vi "DeltaToWye_src.vi"(0 "AB":sgl, 5 "BC":sgl, 7 "CA":sgl) -> (4 "A":sgl, 6 "B":sgl, 8 "C":sgl)   [LabVIEW 2015]
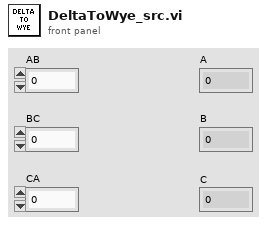
[diagram p1: front panel]
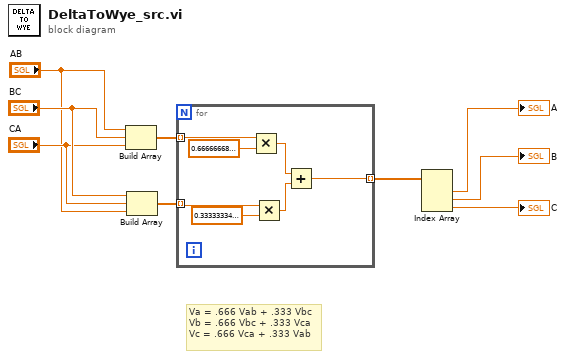
[diagram p0: block diagram]
diagram:
  # "Va = .666 Vab + .333 Vbc\nVb = .666 Vbc + .333 Vca\nVc = .666 Vca + .333 Vab"
  n1 = Build Array("AB", "BC", "CA") -> (w6:sgl[])
  n2 = Build Array("BC", "CA", "AB") -> (w5:sgl[])
  n3 = for {
    tunnel: w6 -> [w16] mode=indexing
    tunnel: w5 -> [w13] mode=indexing
    tunnel: [w10] -> w4 mode=indexing
    n4 = Multiply(x=w16, y=sgl 0.6666667) -> (x*y=w12:sgl)
    n5 = Multiply(x=w13, y=sgl 0.33333334) -> (x*y=w11:sgl)
    n6 = Add(x=w12, y=w11) -> (x+y=w10:sgl)
  }
  n7 = Index Array(array=w4) -> (element #1=→"A":sgl, element #2=→"B":sgl, element #3=→"C":sgl)  [unwired: 3 in]
